vi "Initialize.vi"(0 "VISA resource name":refnum<visa-resource-name>="COM1", 5 "Serial Configuration":T1={"Baud Rate"=9600, "Parity"=0, "Data Bits"=8, "Stop Bits"=10, "Flow Control"=0} {"Flow Control" items=["None", "XON/XOFF", "RTS/CTS", "XON/XOFF & RTS/CTS", "DTR/DSR", "XON/XOFF & DTR/DSR"]; "Stop Bits" items=["1.0"=10, "1.5"=15, "2.0"=20]; "Data Bits" items=["7"=7, "8"=8]; "Parity" items=["None", "Odd", "Even", "Mark", "Space"]; "Baud Rate" items=["300"=300, "600"=600, "1200"=1200, "2400"=2400, "4800"=4800, "9600"=9600, "19200"=19200]}, 9 "Reset (True)":bool=TRUE, 11 "error in (no error)":errorcluster, 12 "Timeout (10000 ms)":u32=10000) -> (4 "VISA resource name out":refnum<visa-resource-name>, 15 "error out":errorcluster)   [LabVIEW 2020, in "eec 6700.lvlib"]
doc: "Establishes communication with the instrument and optionally performs an instrument identification query and/or an instrument reset. It also places the instrument in a default state needed for other instrument driver operations. Therefore, call this VI before calling other instrument driver VIs for this instrument. Generally, you need to call the Initialize VI only once at the beginning of an application."
uses:
  <instrlib>/eec 6700/eec 6700.lvlib
  <instrlib>/eec 6700/Private/Extended User Data.ctl
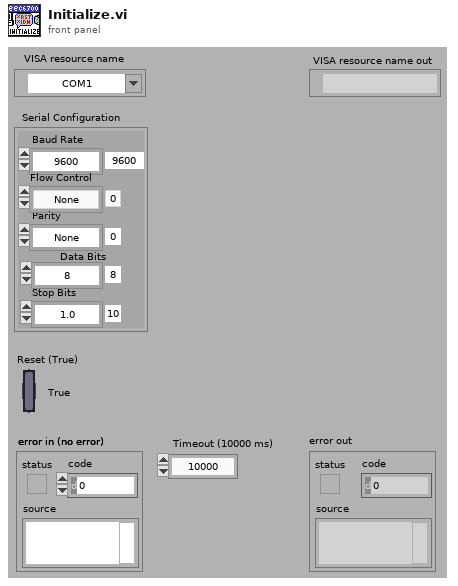
[diagram p1: front panel]
types:
  T1 = cluster{"Baud Rate":u32, "Parity":u16, "Data Bits":u16, "Stop Bits":u16, "Flow Control":u16}
  T2 = typedef "eec 6700.lvlib/Extended User Data.ctl" = cluster{"Firmware Version":string, "eec Models":enum16{"6605", "6610", "6620", "6630", "6650"}}
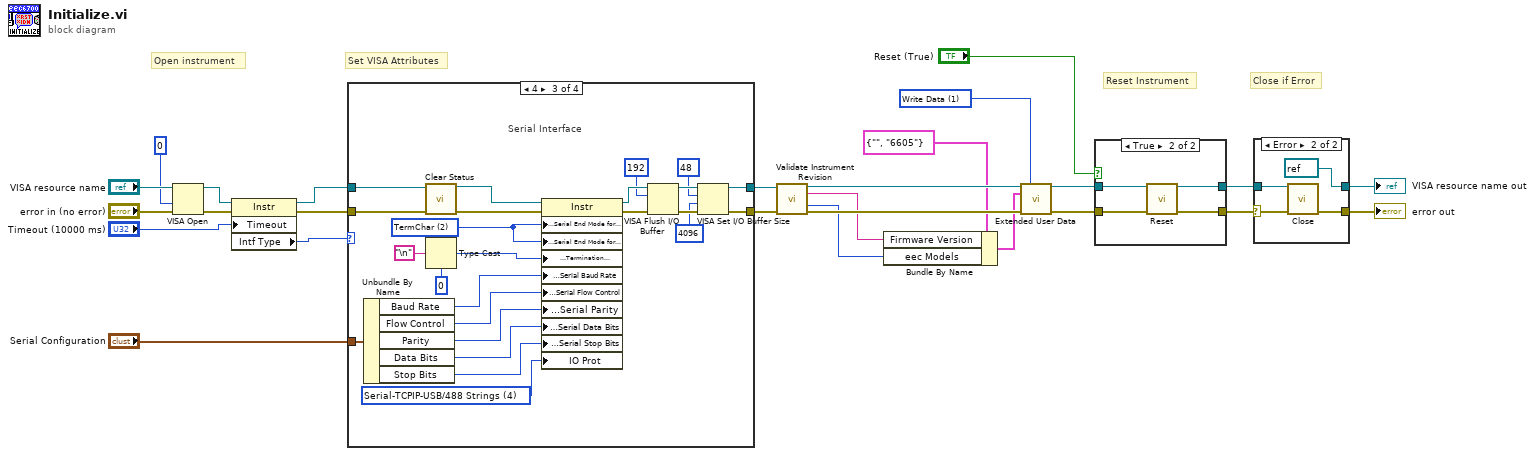
[diagram p0: block diagram]
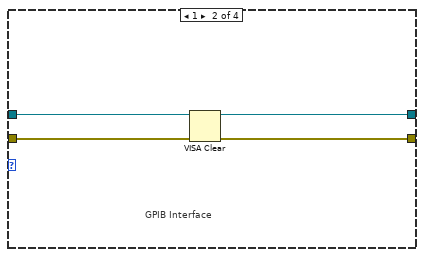
[diagram p3: hidden frame]
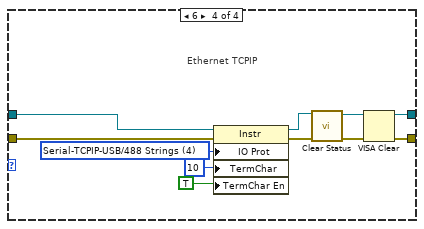
[diagram p4: hidden frame]
diagram:
  w12 = u16 1 items=["Read Data", "Write Data", "Clear Data", "Clear ALL Data"] ("Action")
  # "Set VISA Attributes"
  # "Close if Error"
  # "Reset Instrument"
  # "Open instrument"
  n1 = VISA Open(access mode=u32 0, error in (no error)="error in (no error)", VISA resource name="VISA resource name") -> (VISA resource name=w21:refnum<visa-resource-name>, error out=w20:errorcluster)  [unwired: 2 in]
  n2 = property on="Property Node" class="Instr"(reference=w21, error in=w20, "Timeout"="Timeout (10000 ms)") -> (reference out=w11:refnum<visa-resource-name>, error out=w10:errorcluster, "Intf Type"=w9:u16)
  n3 = case shown="4" w9 {
    tunnel: [w28 w31 w56 w59] -> w23
    tunnel: [w27 w32 w54 w58] -> w22
    tunnel: w11 -> [w28 w29 w35 w67]
    tunnel: w10 -> [w27 w30 w36 w63]
    tunnel: "Serial Configuration" -> [_ _ w43 _]
    frame Default {
    }
    frame 1 {
      # "GPIB Interface"
      n4 = VISA Clear(VISA resource name=w29, error in (no error)=w30) -> (VISA resource name out=w31:refnum<visa-resource-name>, error out=w32:errorcluster)
    }
    frame 4 {
      w37 = u16 4 items=["Normal"=1, "VXI/FDC"=2, "GPIB/HS488"=3, "Serial-TCPIP-USB/488 Strings"=4, "USBTMC/Vendor-Specific"=5] ("Message Based Settings:IO Protocol")
      w50 = u16 2 items=["None", "LastBit", "TermChar"] ("Serial Settings:Serial End Mode for Reads")
      # "Serial Interface"
      n5 = Unbundle By Name(w43) -> ("Baud Rate"=w48:u32, "Flow Control"=w45:u16, "Parity"=w46:u16, "Data Bits"=w47:u16, "Stop Bits"=w44:u16)
      n6 = call <instrlib>:"Clear Status.vi"("VISA resource name"=w35, "error in (no error)"=w36) -> ("VISA resource name out"=w34:refnum<visa-resource-name>, "error out"=w33:errorcluster)  [unwired: 12 in]
      n7 = Type Cast(type=u8 0, x="\n" ("Line Feed Constant")) -> (*(type *) &x=w49:u8)
      n8 = property on="Property Node" class="Instr"(reference=w34, error in=w33, "Serial Settings:Serial End Mode for Reads"=w50, "Serial Settings:Serial End Mode for Writes"=w50, "Message Based Settings:Termination Character"=w49, "Serial Settings:Serial Baud Rate"=w48, "Serial Settings:Serial Flow Control"=w45, "Serial Settings:Serial Parity"=w46, "Serial Settings:Serial Data Bits"=w47, "Serial Settings:Serial Stop Bits"=w44, "IO Prot"=w37) -> (reference out=w53:refnum<visa-resource-name>, error out=w55:errorcluster)
      n9 = VISA Flush I/O Buffer(VISA resource name=w53, mask (16)=u16 192, error in (no error)=w55) -> (VISA resource name out=w42:refnum<visa-resource-name>, error out=w41:errorcluster)
      n10 = VISA Set I/O Buffer Size(VISA resource name=w42, mask (16)=u16 48, size (4096)=u32 4096 ("size (0)"), error in (no error)=w41) -> (VISA resource name out=w56:refnum<visa-resource-name>, error out=w54:errorcluster)
    }
    frame 6 {
      w66 = u16 4 items=["Normal"=1, "VXI/FDC"=2, "GPIB/HS488"=3, "Serial-TCPIP-USB/488 Strings"=4, "USBTMC/Vendor-Specific"=5] ("Message Based Settings:IO Protocol")
      # "Ethernet TCPIP"
      n11 = property on="Property Node" class="Instr"(reference=w67, error in=w63, "IO Prot"=w66, "TermChar"=u8 10 ("Message Based Settings:Termination Character"), "TermChar En"=TRUE ("Message Based Settings:Termination Character Enable")) -> (reference out=w61:refnum<visa-resource-name>, error out=w62:errorcluster)
      n12 = call <instrlib>:"Clear Status.vi"("VISA resource name"=w61, "error in (no error)"=w62) -> ("VISA resource name out"=w57:refnum<visa-resource-name>, "error out"=w60:errorcluster)  [unwired: 12 in]
      n13 = VISA Clear(VISA resource name=w57, error in (no error)=w60) -> (VISA resource name out=w59:refnum<visa-resource-name>, error out=w58:errorcluster)
    }
  }
  n14 = call <instrlib>:"Validate Instrument Revision.vi"("VISA resource name"=w23, "error in (no error)"=w22) -> ("VISA resource name out"=w8:refnum<visa-resource-name>, "Firmware Version"=w3:string, "Model Number"=w4:enum16{"6605", "6610", "6620", "6630", "6650"}, "error out"=w7:errorcluster)  [unwired: 10 in]
  n15 = Bundle By Name(cluster=T2 {"Firmware Version"="", "eec Models"=enum."6605"} ("User Data In"), "Firmware Version"=w3, "eec Models"=w4) -> (w6:T2)
  n16 = call <instrlib>:"Extended User Data.vi"("VISA resource name"=w8, "Action"=w12, "User Data In"=w6, "Error In (no error)"=w7) -> ("VISA resource name out"=w14:refnum<visa-resource-name>, "Error Out"=w13:errorcluster)  [unwired: 9 in, 1 out]
  n17 = case shown="True" "Reset (True)" {
    tunnel: w13 -> [w68 w70]
    tunnel: [w68 w72] -> w2
    tunnel: w14 -> [w69 w71]
    tunnel: [w69 w73] -> w17
    frame False {
    }
    frame True {
      n18 = call <instrlib>:"Reset.vi"("VISA resource name"=w71, "error in (no error)"=w70) -> ("VISA resource name out"=w73:refnum<visa-resource-name>, "error out"=w72:errorcluster)  [unwired: 12 in]
    }
  }
  n19 = case shown="Error" w2 {
    selector: w2 -> [w74 w77]
    tunnel: w17 -> [w75 w78]
    tunnel: [w75 refnum<visa-resource-name> refnum ("VISA resource name out")] -> w19
    tunnel: [w74 w79] -> w18
    frame No Error {
    }
    frame Error {
      n20 = call <instrlib>:"Close.vi"("VISA resource name"=w78, "error in (no error)"=w77) -> ("error out"=w79:errorcluster)  [unwired: 13 in]
    }
  }
  "VISA resource name out" <- w19
  "error out" <- w18
